vi "Open Word File_ActiveX 2012.vi"() -> ()   [LabVIEW 2017]
doc: "This example shows how to open word file using ActiveX control."
panel:
  in  "Exit":bool
  in  "Open File":bool
  out "Quit":bool
  in  "error in (no error)":errorcluster
  out "error out":errorcluster
  in  "Word File":path
  # "Overview: This example shows how to open word file using ActiveX control.\nRequirements: LabVIEW 2012 (or compatible)\nInstructions:\n1. Run the VI.\n2. Specify the path of Word File.\n3. Click on the Open File button to open the word file."
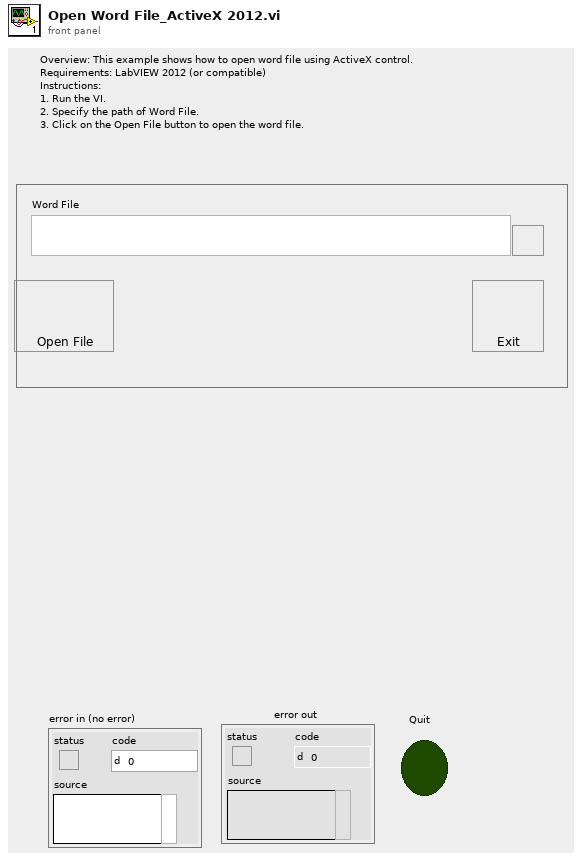
[diagram p1: front panel]
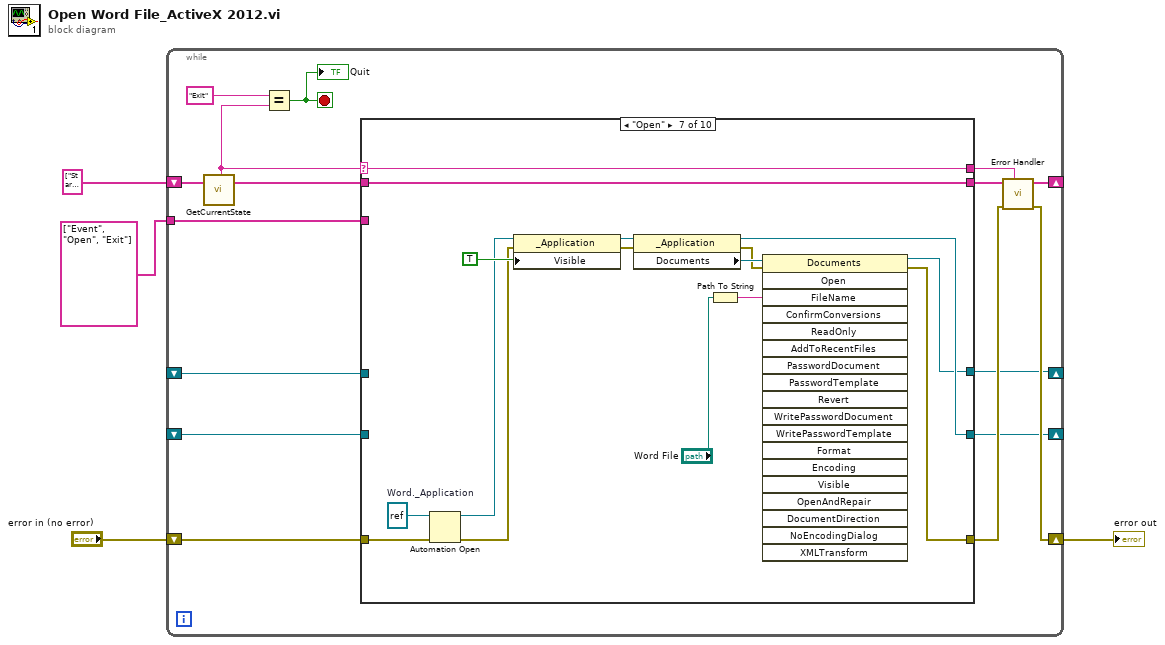
[diagram p0: block diagram]
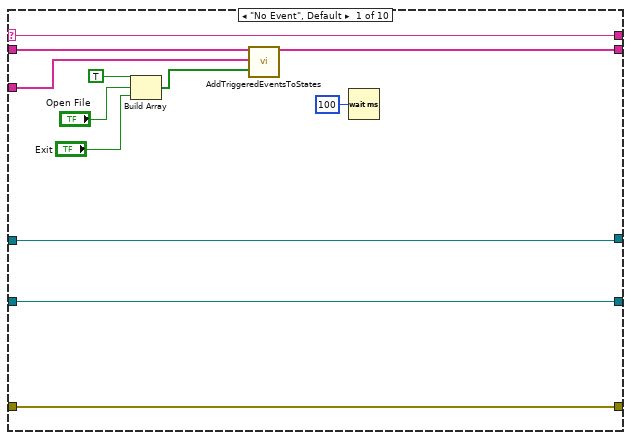
[diagram p2: hidden frame]
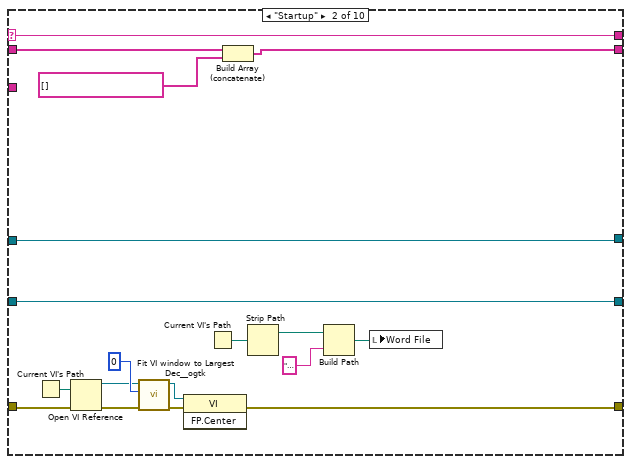
[diagram p3: hidden frame]
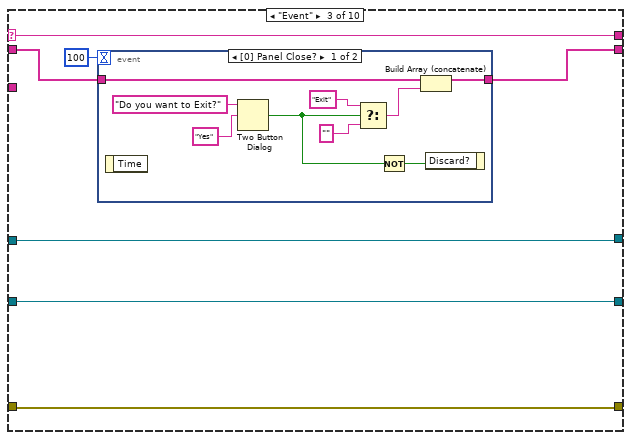
[diagram p4: hidden frame]
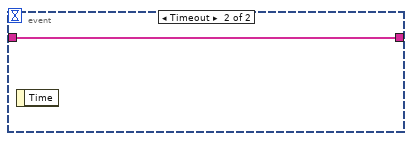
[diagram p5: hidden frame]
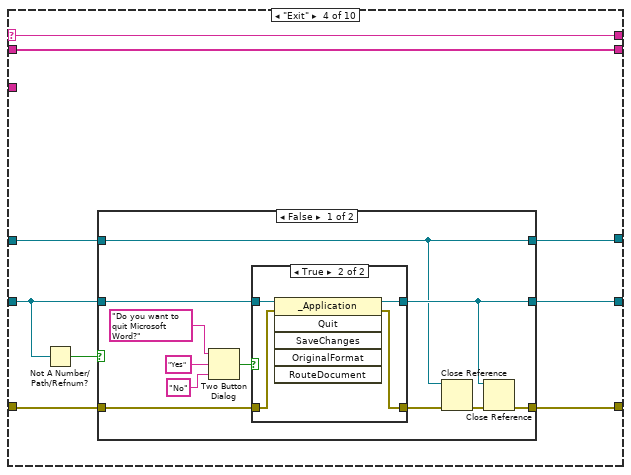
[diagram p6: hidden frame]
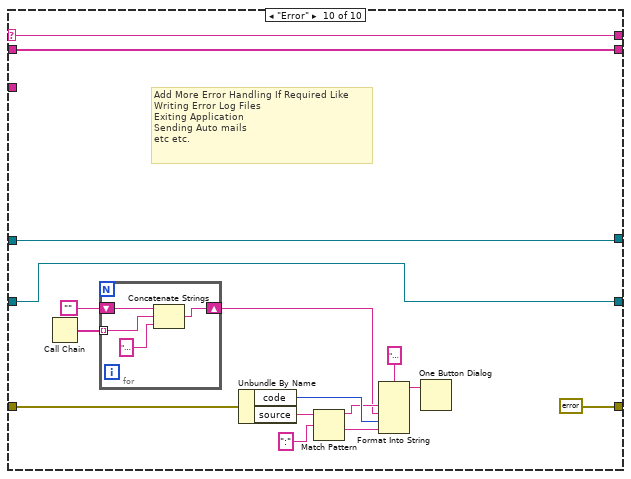
[diagram p13: hidden frame]
diagram:
  n1 = while {
    shift-right: [w13] -> _
    shift-left: string[] ["Startup"] ("State Array Out") -> [w20]
    tunnel: string[] ["Event", "Open", "Exit"] ("State Array Out") -> [w18]
    shift-right: [w10] -> w3
    shift-left: "error in (no error)" -> [w14]
    shift-right: [w8] -> _
    shift-left: _ -> [w7]
    shift-right: [w6] -> _
    shift-left: _ -> [w5]
    stop <- w15 stop-if-true
    n2 = call "GetCurrentState.vi"("State Array In"=w20) -> ("Current State"=w16:string, "State Array Out"=w19:string[])  [unwired: 1 in, 16 out]
    n3 = Equal?(x="Exit", y=w16) -> (x = y?=w15:bool)
    "Quit" <- w15
    n4 = case shown="\"Open\"" w16 {
      selector: w16 -> [w28 w47 w57 w76 w99 w104 w122 w125 w132 w148]
      tunnel: w19 -> [w32 w49 w55 w75 w101 w106 w111 w127 w131 w147]
      tunnel: [w25 w48 w54 w75 w101 w106 w111 w127 w131 w147] -> w12
      tunnel: w18 -> [w31 _ _ _ _ _ _ _ _ _]
      tunnel: [w29 w33 w56 w74 w100 w105 w108 w126 w130 errorcluster {"status"=FALSE, "code"=0, "source"=""} ("error in (no error)")] -> w9
      tunnel: w14 -> [w29 w41 w56 w73 w100 w105 w107 w126 w130 w146]
      tunnel: [w28 w47 w57 w76 w99 w104 w122 w125 w132 w148] -> w11
      tunnel: [w24 w34 w53 w72 w98 w102 w115 w124 w129 w134] -> w8
      tunnel: w7 -> [w24 w34 w53 w71 w98 w102 _ w124 w129 w134]
      tunnel: [w22 w39 w52 w68 w97 w103 w114 w123 w128 w133] -> w6
      tunnel: w5 -> [w22 w39 w52 w69 w97 w103 _ w123 w128 w133]
      frame "No Event", Default {
        n5 = Build Array(TRUE, "Open File", "Exit") -> (w27:bool[])
        n6 = call "AddTriggeredEventsToStates.vi"("State Array In"=w32, "Event List"=w31, "Event Triggers Array"=w27) -> ("State Array Out"=w25:string[])  [unwired: 16 out]
        n7 = Wait (ms)(milliseconds to wait=u32 100 ("millisecond multiple")) -> ()  [unwired: 1 out]
      }
      frame "Startup" {
        n8 = Current VI's Path() -> (path=w44:path)
        n9 = Open VI Reference(vi path=w44, error in (no error)=w41) -> (vi reference=w45:refnum<vi>, error out=w40:errorcluster)  [unwired: 4 out]
        n10 = call "Fit VI window to Largest Dec__ogtk.vi"("error in (no error)"=w40, "border spacing (2 px)"=0, "VI Ref (calling VI)"=w45) -> ("error out"=w43:errorcluster, "dup VI Ref"=w42:refnum<vi>)  [unwired: 3 out]
        n11 = invoke class="VI" method="FP.Center"(reference=w42, error in=w43) -> (error out=w33:errorcluster)  [unwired: 1 in, 2 out]
        n12 = Current VI's Path() -> (path=w38:path)
        n13 = Build Array (concatenate)(w49, string[] [] ("State Array Out")) -> (w48:string[])
        n14 = Strip Path(path=w38) -> (stripped path=w37:path)  [unwired: 1 out]
        n15 = Build Path(base path=w37, name or relative path="Test.doc") -> (appended path=w35:path)
        n16 = local write "Word File"(w35) -> ()
      }
      frame "Event" {
        n17 = event shown="[0] Panel Close?" {
          selector: _ -> [_ _]
          dyn-events: _ -> [_ _]
          timeout: 100 -> [_ _]
          tunnel: w55 -> [w66 w67]
          tunnel: [w62 w67] -> w54
          event Panel Close? {
            n18 = event-data() -> ()  [unwired: 1 in, 1 out]
            n19 = Two Button Dialog(message="Do you want to Exit?", 2:"Yes" ("T button name (\"OK\")")) -> (T button?=w61:bool)  [unwired: 1 in]
            n20 = Select(t="Exit" ("x"), s=w61, f="") -> (s? t:f=w59:string)
            n21 = Not(x=w61) -> (.not. x?=w63:bool)
            n22 = Build Array (concatenate)(w66, w59) -> (w62:string[])
            n23 = event-data("Discard?"=w63) -> ()  [unwired: 1 in, 1 out]
          }
          event Timeout {
            n24 = event-data() -> ()  [unwired: 1 in, 1 out]
          }
        }
      }
      frame "Exit" {
        n25 = Not A Number/Path/Refnum?(number/path/refnum=w71) -> (NaN/Path/Refnum?=w70:bool)
        n26 = case shown="False" w70 {
          tunnel: [w87 w95] -> w74
          tunnel: w73 -> [w82 w95]
          tunnel: w71 -> [w80 w96]
          tunnel: [w79 w96] -> w72
          tunnel: w69 -> [w77 w94]
          tunnel: [w77 w94] -> w68
          frame False {
            n27 = Two Button Dialog(message="Do you want to quit Microsoft Word?", 1:"No" ("F button name (\"Cancel\")"), 2:"Yes" ("T button name (\"OK\")")) -> (T button?=w83:bool)
            n28 = case shown="True" w83 {
              tunnel: w80 -> [w88 w93]
              tunnel: w82 -> [w89 w92]
              tunnel: [w89 w91] -> w81
              tunnel: [w88 w90] -> w79
              frame False {
              }
              frame True {
                n29 = invoke class="_Application" method="Quit"(reference=w93, error in=w92) -> (reference out=w90:refnum<k7>, error out=w91:errorcluster)  [unwired: 4 in, 4 out]
              }
            }
            n30 = Close Reference(reference=w77, error in (no error)=w81) -> (error out=w78:errorcluster)
            n31 = Close Reference(reference=w79, error in (no error)=w78) -> (error out=w87:errorcluster)
          }
          frame True {
          }
        }
      }
      frame "---------------Below are UI Events---------------" {
      }
      frame "Print" {
      }
      frame "Open" {
        w113 = refnum<k7> refnum  # Word._Application
        n32 = Automation Open(error in (no error)=w107, Automation Refnum=w113) -> (Automation Refnum=w112:refnum<k7>, error out=w109:errorcluster)  [unwired: 2 in]
        n33 = property class="_Application"(reference=w112, error in=w109, "Visible"=TRUE) -> (reference out=w121:refnum<k7>, error out=w120:errorcluster)
        n34 = property class="_Application"(reference=w121, error in=w120) -> (reference out=w115:refnum<k7>, error out=w110:errorcluster, "Documents"=w117:refnum<k7>)
        n35 = Path To String(path="Word File") -> (string=w118:string)
        n36 = invoke class="Documents" method="Open"(reference=w117, error in=w110, "FileName"=w118) -> (reference out=w114:refnum<k7>, error out=w108:errorcluster)  [unwired: 16 in, 17 out]
      }
      frame "---------------Below are Subroutine states---------------" {
      }
      frame "---------------Below are Error Handling VIs---------------" {
      }
      frame "Error" {
        # "Add More Error Handling If Required Like\nWriting Error Log Files\nExiting Application\nSending Auto mails\netc etc."
        n37 = Call Chain() -> (call chain=w139:string[])
        n38 = for {
          tunnel: w139 -> [w151] mode=indexing
          shift-right: [w149] -> w136
          shift-left: "" -> [w152]
          n39 = Concatenate Strings(w152, w151, " -> ") -> (w149:string)
        }
        n40 = Unbundle By Name(w146) -> ("code"=w141:i32, "source"=w144:string)
        n41 = Match Pattern(string=w144, regular expression=":") -> (before substring=w137:string, after substring=w142:string)  [unwired: 3 out]
        n42 = Format Into String(format string="Error Occured In\"%s\" state of \"%s\" VI\nError Code: %d\nError Description: \"%s\"", w137, w136, w141, w142) -> (resulting string=w140:string)  [unwired: 2 in, 1 out]
        n43 = One Button Dialog(message=w140) -> ()  [unwired: 2 out]
      }
    }
    n44 = call "Error Handler.vi"("Current State"=w11, "error in (no error)"=w9, "Msg Queue In"=w12) -> ("error out"=w10:errorcluster, "Msg Queue Out"=w13:string[])  [unwired: 7 out]
  }
  "error out" <- w3
